vi "HELP.vi"(8 "error in (no error)":errorcluster, 11 "Instrument in":refnum<class "Instrument.lvclass">) -> (0 "error out":errorcluster, 2 "Commands":string[](array[string]), 3 "Instrument in":refnum<class "Instrument.lvclass">)   [LabVIEW 2019, in "Instrument.lvclass"]
doc: "Send \"HELP\" command to get API supported by remote Instrument."
uses:
  Instrument.lvclass
  Typedefs/Instrument.Commands--Enum.ctl
  df6d36b1-df84-4a1a-80e3-72715317c370.vi
  df6d36b1-df84-4a1a-80e3-72715317c370.vi/719754d3-54fd-4c68-af66-58aa178a4cc8.vi
  df6d36b1-df84-4a1a-80e3-72715317c370.vi/66edb4b2-e370-4814-b1f5-ffbe2ca3155b.vi
  <vilib>/Utility/Data Type/Get Type Information.vi
  <vilib>/JDP Science/JSONtext/JSON text to Variant.vi
  <vilib>/JDP Science/JSONtext/LVClass Serializer/JSONtext LVClass Serializer.lvclass
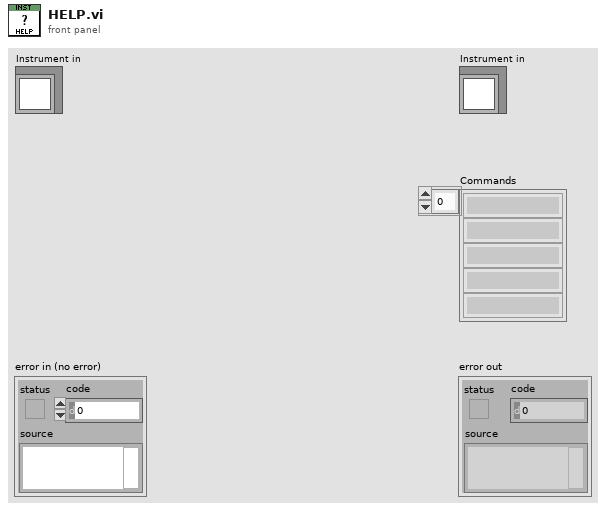
[diagram p1: front panel]
types:
  T1 = typedef "Instrument.lvclass/Instrument.Commands--Enum.ctl" = enum16{"ACK", "HELP", "setConfiguration", "setLogData", "getAll", "getAllData"}
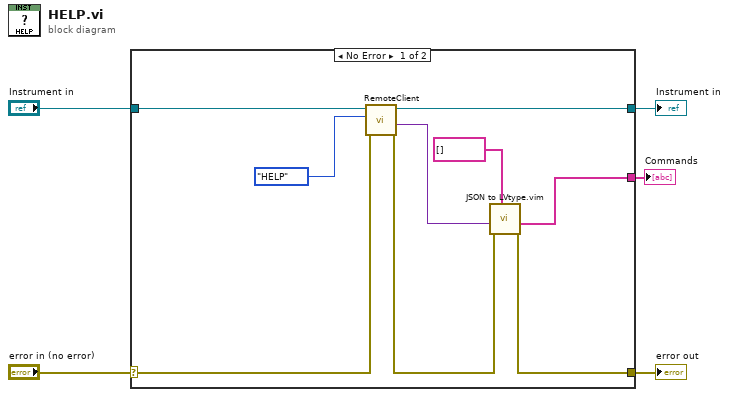
[diagram p0: block diagram]
diagram:
  n1 = case shown="No Error" "error in (no error)" {
    selector: "error in (no error)" -> [w12 w16]
    tunnel: [w8 w16] -> w4
    tunnel: [w14 w15] -> w2
    tunnel: "Instrument in" -> [w13 w15]
    tunnel: [w6 _] -> w1
    frame No Error {
      n2 = call "RemoteClient.vi"("error in (no error)"=w12, "Command in"=Instrument.Commands--Enum."HELP" ("Commands"), "Instrument in"=w13) -> ("error out"=w9:errorcluster, "Data out"=w7:variant, "Instrument out"=w14:refnum<class "Instrument.lvclass">)  [unwired: 5 in, 1 out]
      n3 = call "JSON to LVtype.vim"("type"=string[] [] ("Commands"), "error in (no error)"=w9, "JSON Data in"=w7) -> ("error out"=w8:errorcluster, "Data out"=w6:string[])  [unwired: 7 in]
    }
    frame Error {
    }
  }
  "error out" <- w4
  "Instrument in" <- w2
  "Commands" <- w1
